vi "FlatToRichni_measurementlink_discovery_v1_UnregisterServiceResponse.vi"(5 "OutputClusterType":T1, 11 "InputCluster":T2) -> (3 "OutputCluster":T1)   [LabVIEW 2021, in "ni.measurementlink.discovery.v1.api.lvlib"]
uses:
  ni.measurementlink.discovery.v1.api.lvlib
  ni_measurementlink_discovery_v1_UnregisterServiceResponse_Flat.ctl
  ni_measurementlink_discovery_v1_UnregisterServiceResponse.ctl
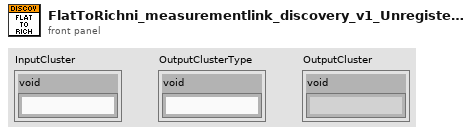
[diagram p1: front panel]
types:
  T1 = typedef "ni.measurementlink.discovery.v1.api.lvlib/ni_measurementlink_discovery_v1_UnregisterServiceResponse.ctl" = cluster{"void":string}
  T2 = typedef "ni.measurementlink.discovery.v1.api.lvlib/ni_measurementlink_discovery_v1_UnregisterServiceResponse_Flat.ctl" = cluster{"void":string}
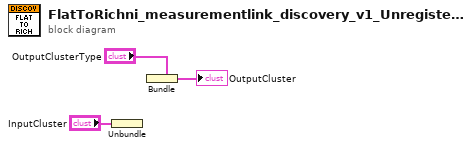
[diagram p0: block diagram]
diagram:
  n1 = Unbundle "Unbundle"("InputCluster") -> ()  [unwired: 1 out]
  n2 = Bundle "Bundle"(cluster="OutputClusterType") -> (→"OutputCluster":T1)  [unwired: 1 in]
